vi "trace_idxVacant.vi"(9 "idx start":i32, 11 "traces active":u64 format="%b") -> (0 "none free":bool, 1 "idx free":i32, 3 "traces active out":u64 format="%b")   [LabVIEW 2010, in "OSA.lvclass"]
uses:
  OSA.lvclass
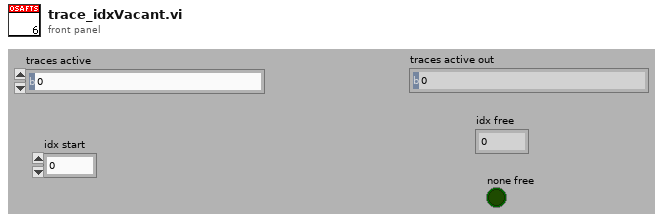
[diagram p1: front panel]
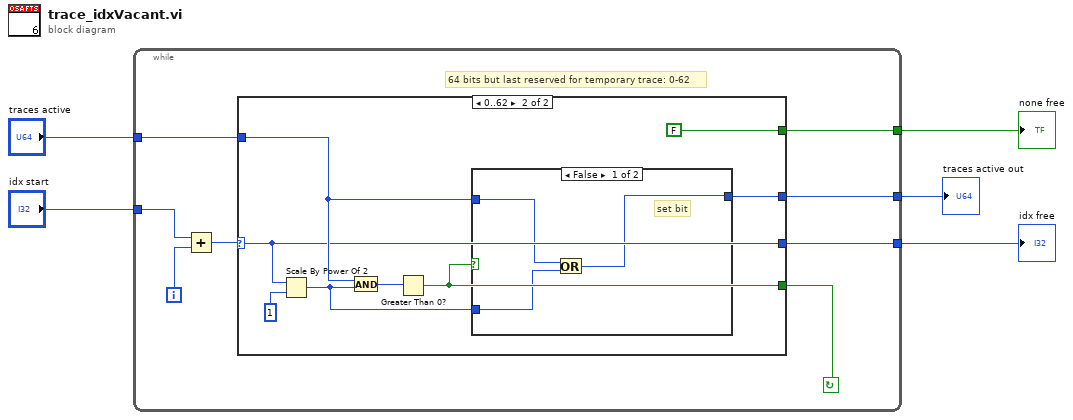
[diagram p0: block diagram]
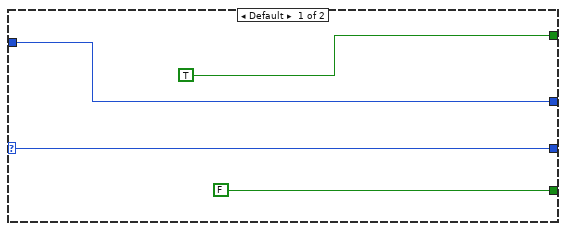
[diagram p2: hidden frame]
diagram:
  n1 = while {
    tunnel: "traces active" -> [w13]
    tunnel: "idx start" -> [w9]
    tunnel: [w8] -> w3
    tunnel: [w7] -> w2
    tunnel: [w6] -> w1
    i -> [w12]
    stop <- w10 continue-if-true
    # "64 bits but last reserved for temporary trace: 0-62"
    n2 = Add(x=w9, y=w12) -> (x+y=w11:i32)
    n3 = case shown="0..62" w11 {
      selector: w11 -> [w16 w20]
      tunnel: w13 -> [w14 w21]
      tunnel: [FALSE w22] -> w10
      tunnel: [w16 w20] -> w8
      tunnel: [TRUE FALSE] -> w7
      tunnel: [w14 w18] -> w6
      frame Default {
      }
      frame 0..62 {
        n4 = Scale By Power Of 2(n=w20, x=u64 1) -> (x*2^n=w19:u64)
        n5 = And(x=w21, y=w19) -> (x .and. y?=w24:u64)
        n6 = Greater Than 0?(x=w24) -> (x > 0?=w22:bool)
        n7 = case shown="False" w22 {
          tunnel: w21 -> [w28 w29]
          tunnel: w19 -> [w27 _]
          tunnel: [w26 w29] -> w18
          frame False {
            # "set bit"
            n8 = Or(x=w28, y=w27) -> (x .or. y?=w26:u64)
          }
          frame True {
          }
        }
      }
    }
  }
  "none free" <- w2
  "idx free" <- w3
  "traces active out" <- w1
